vi "target.vi"() -> ()   [LabVIEW 2020]
uses:
  <vilib>/rvi/interface/RandomDataEmulation/niFpgaRandomDataHandleErrors.vi
  <vilib>/rvi/DataTransferAndStorage/Container/XNode/niFpgaContainer.xnode
  <vilib>/rvi/interface/RandomDataEmulation/nirviRandomDataFpgaReadWriteTemplate.vi
panel:
  out "tick count":u32
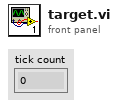
[diagram p1: front panel]
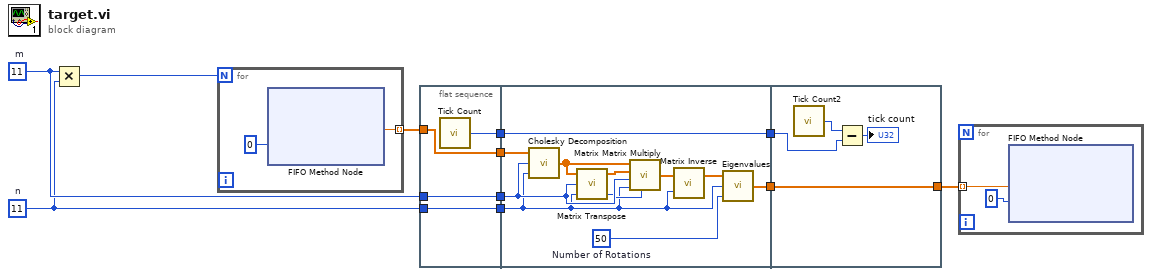
[diagram p0: block diagram]
diagram:
  w7 = 11  # n
  w9 = 11  # m
  n1 = Multiply(x=w9, y=w7) -> (x*y=w11:i32)
  n2 = for {
    N: w11 -> [_]
    tunnel: [w13] -> w10 mode=indexing
    n3 = xnode ("FIFO Method Node")("Timeout"=0) -> ("Element"=w13:sgl)  [unwired: 1 in, 2 out]
  }
  n4 = flat-sequence {
    tunnel: w7 -> [w15]
    tunnel: w9 -> [w16]
    tunnel: w10 -> [w17]
    tunnel: [w17] -> w6
    tunnel: [w16] -> w5
    tunnel: [w15] -> w4
    tunnel: [w14] -> w2
    tunnel: w6 -> [w28]
    tunnel: w5 -> [w27]
    tunnel: w4 -> [w19]
    tunnel: [w20] -> w3
    tunnel: w2 -> [w18]
    tunnel: [w18] -> w1
    tunnel: [w32] -> w8
    tunnel: w3 -> [w32]
    tunnel: w1 -> [w30]
    frame #0 {
      n5 = call "Tick Count"() -> ("Tick Count(Ticks)"=w14:u32)
    }
    frame #1 {
      w21 = 50  # Number of Rotations
      n6 = call <vilib>:"Cholesky Decomposition.vi"("n"=w19, "m"=w27, "A"=w28) -> ("L"=w26:sgl[])
      n7 = call <vilib>:"Matrix Transpose.vi"("n"=w19, "m"=w27, "A"=w26) -> ("n"=w24:i32, "B"=w25:sgl[])  [unwired: 1 out]
      n8 = call <vilib>:"Matrix Matrix Multiply.vi"("p"=w24, "n"=w19, "m"=w27, "B"=w25, "A"=w26) -> ("C"=w23:sgl[])  [unwired: 1 in]
      n9 = call <vilib>:"Matrix Inverse.vi"("n"=w19, "A"=w23) -> ("inv(A)"=w22:sgl[])  [unwired: 1 out]
      n10 = call <vilib>:"Eigenvalues.vi"("Number of Rotations (100)"=w21, "n"=w19, "A"=w22) -> ("eigenvalues"=w20:sgl[])
    }
    frame #2 {
      n11 = call "Tick Count2"() -> ("Tick Count(Ticks)"=w31:u32)
      n12 = Subtract(x=w31, y=w30) -> (x-y=→"tick count":u32)
    }
  }
  n13 = for {
    tunnel: w8 -> [w33] mode=indexing
    n14 = xnode ("FIFO Method Node")("Element"=w33, "Timeout"=0) -> ()  [unwired: 1 in, 2 out]
  }
